vi "Set Parameter Scaling.vi"(8 "error in":errorcluster, 9 "scale offset":dbl, 10 "scale multiplier":dbl=1.0, 11 "parameter ref in":T1 format="%.0x") -> (0 "error out":errorcluster, 3 "parameter ref out":T1 format="%.0x")   [LabVIEW 2020, in "Ballard ARINC 429 Scripting.lvlib"]
uses:
  Ballard ARINC 429 Scripting.lvlib
  <vilib>/NI VeriStand/Custom Device API/Custom Device Item Ref.ctl
  Constants.vi
  <vilib>/NI VeriStand/Custom Device API/Set Item Property (Double).vi
  <vilib>/NI VeriStand/Custom Device API/Custom Device API.lvlib
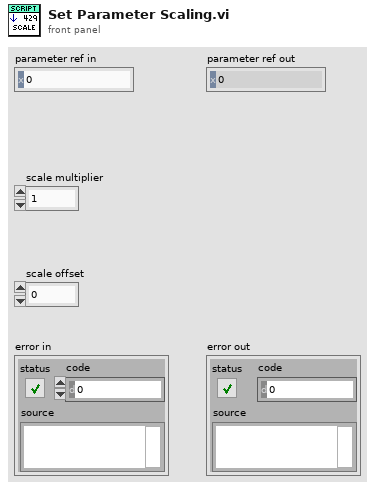
[diagram p1: front panel]
types:
  T1 = typedef "Custom Device API.lvlib/Custom Device Item Ref.ctl" = u64
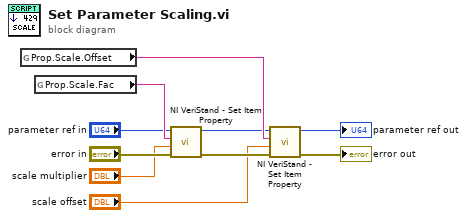
[diagram p0: block diagram]
diagram:
  n1 = global read "Constants.vi" "Prop.Scale.Offset"() -> (w10:string)
  n2 = global read "Constants.vi" "Prop.Scale.Fac"() -> (w9:string)
  n3 = call-poly <vilib>:"NI VeriStand - Set Item Property.vi"("error in (no error)"="error in", "Value"="scale multiplier", "Property Name"=w9, "Item Ref in"="parameter ref in") -> ("error out"=w6:errorcluster, "Item Ref out"=w3:T1)  [unwired: 5 in, 1 out]
  n4 = call-poly <vilib>:"NI VeriStand - Set Item Property.vi"("error in (no error)"=w6, "Value"="scale offset", "Property Name"=w10, "Item Ref in"=w3) -> ("error out"=→"error out":errorcluster, "Item Ref out"=→"parameter ref out":T1)  [unwired: 5 in, 1 out]
